vi "Filter Tree Item Close Event.vi"(8 "error in (no error)":errorcluster, 10 "TreeItemCloseMsg":refnum<class "TreeItemCloseMsg.lvclass">, 11 "IEventFilter in":refnum<class "IEventFilter.lvclass">) -> (0 "error out":errorcluster, 1 "Discard?":bool, 3 "IEventFilter out":refnum<class "IEventFilter.lvclass">)   [LabVIEW 2017, in "ActorEvents.lvlib" / "IEventFilter.lvclass"]
uses:
  IEventFilter.lvclass
  IEventAggregator Messages/TreeItemCloseMsg/TreeItemCloseMsg.lvclass
panel:
  # "No additional\nEvent Data"
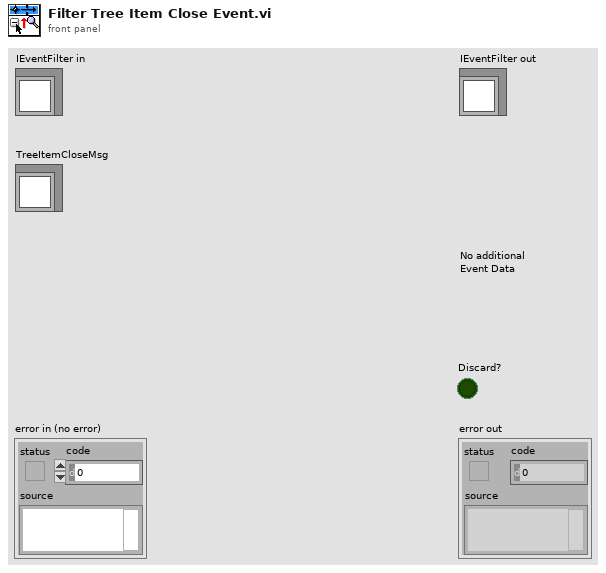
[diagram p1: front panel]
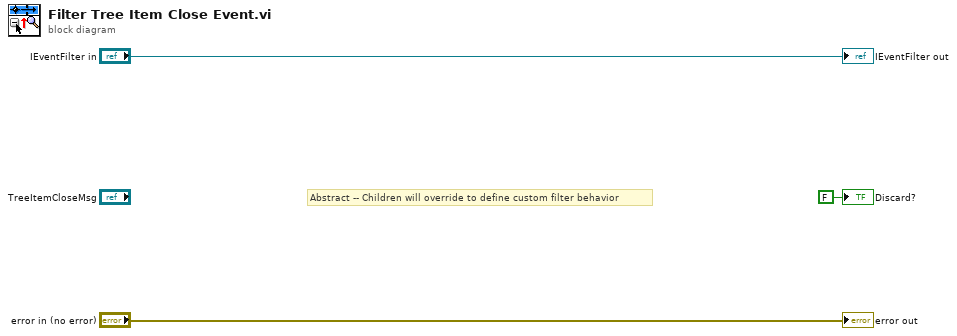
[diagram p0: block diagram]
diagram:
  # "Abstract -- Children will override to define custom filter behavior"
  "error out" <- "error in (no error)"
  "IEventFilter out" <- "IEventFilter in"
  "Discard?" <- FALSE ("Discard?")
